vi "Create Logger.vi"(8 "error in (no error)":errorcluster, 9 "Debug Level (Default)":T1, 10 "Sinks (Default)":refnum<class "Sink.lvclass">[](array[class]), 11 "Name":string) -> (0 "error out":errorcluster, 3 "Logger out":refnum<class "Logger.lvclass">)   [LabVIEW 2020, in "LV Log.lvlib"]
uses:
  LV Log.lvlib
  Logger/Logger.lvclass
  Sink/Sink.lvclass
  Type Defs/Debug Level.ctl
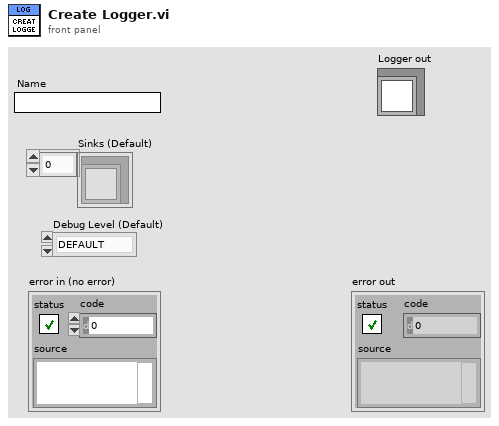
[diagram p1: front panel]
types:
  T1 = typedef "LV Log.lvlib/Debug Level.ctl" = enum16{"DEFAULT", "DEBUG", "INFO", "WARN", "ERROR", "FATAL"}
  T2 = enum16{"Init", "Get Logger", "Register Sink", "Set Global Debug Level", "Get Sinks", "Get Global Debug Level", "Register Logger"}
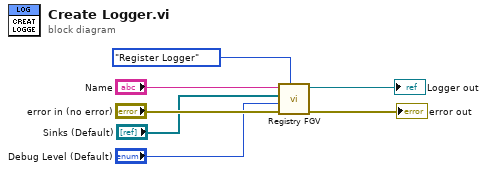
[diagram p0: block diagram]
diagram:
  n1 = call "Registry FGV.vi"("State (Get Logger)"=T2."Register Logger", "error in (no error)"="error in (no error)", "Debug Level in"="Debug Level (Default)", "Sink(s)"="Sinks (Default)", "Name"="Name") -> ("error out"=→"error out":errorcluster, "Logger out"=→"Logger out":refnum<class "Logger.lvclass">)  [unwired: 3 in, 2 out]
